vi "ex05_math_ops_cvt.vi"() -> ()   [LabVIEW 2019]
panel:
  out "number":dbl format="%.2f"
  out "decimal integer string":string
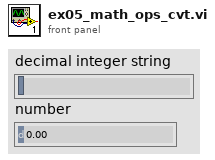
[diagram p1: front panel]
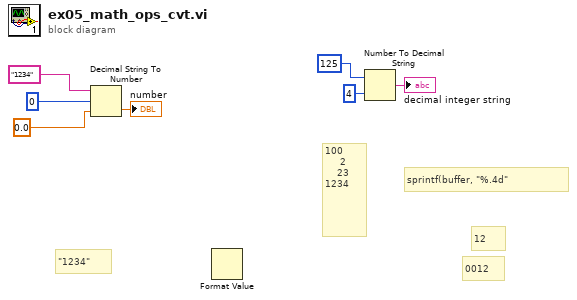
[diagram p0: block diagram]
diagram:
  # "\"1234\""
  # "0012"
  # "12"
  # "sprintf(buffer, \"%.4d\""
  # "100\n     2\n    23\n1234"
  n1 = Decimal String To Number(string="1234", offset=0, default (0L)=0.0) -> (number=→"number":dbl)  [unwired: 1 out]
  n2 = Format Value() -> ()  [unwired: 3 in, 1 out]
  n3 = Number To Decimal String(number=125, width (-)=i16 4) -> (decimal integer string=→"decimal integer string":string)
